vi "界面UI.vi"() -> ()   [LabVIEW 2016, in "科盛超标留样.lvlib"]
uses:
  <vilib>/Utility/miscctls.llb/LVPointTypeDef.ctl
  <vilib>/Utility/config.llb/NI_LVConfig.lvlib
  <vilib>/ptbypt/NI_PtbyPt.lvlib
panel:
  out "开关量3状态":T1
  out "开关量2状态":T2
  out "开关量1状态":T3
  out "元素":enum16{"open", "read", "write", "close"}(ring)
  out "供样完成":bool
  in  "返回":bool
  in  "查看记录":bool
  in  "当前解析模式":string(combo)
  in  "切换串口":bool
  out "查询系统状态":T4
  out "查询瓶记录":T5
  out "输出数组":T6(array[cluster])
  in  "留样命令":bool
  in  "供样命令":bool
  in  "触发采样":bool
  in  "查询系统状态":bool
  in  "远程取样":bool
  in  "复位指令":bool
  in  "查询瓶记录":bool
  in  "查询采样记录":bool
  in  "VISA resource name":refnum<visa-resource-name>="COM2" caption="VISA资源名称"
  in  "写入缓冲区":string
  out "读取缓冲区":string
  out "source":string
  out "通讯":bool
  # "启动顺序：先触发采样，然后仪器开始测试时发送供样命令此时采水到A/B桶，如果超标发送留样命令，如果在默认60分钟(可设置)后都没有接受到超标留样指令则自动排空。"
  # "科盛超标留样"
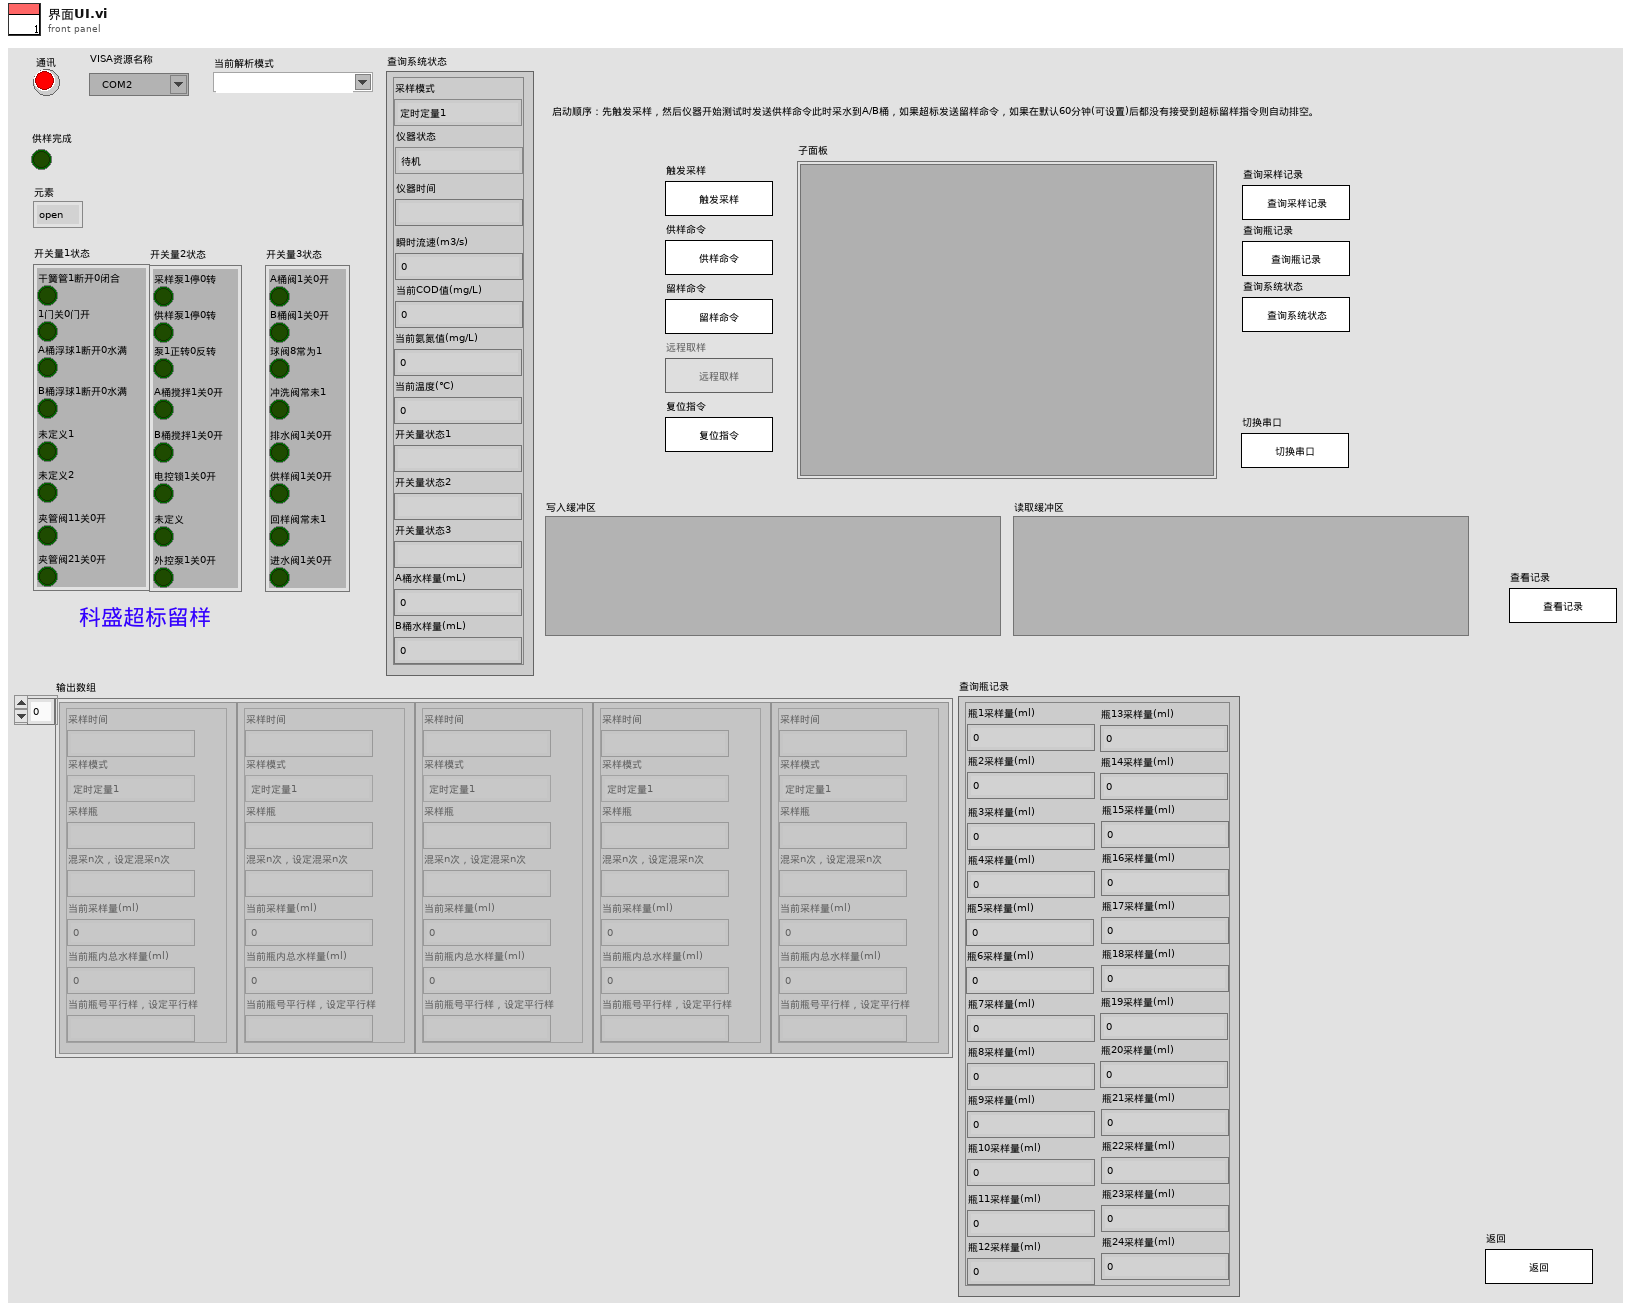
[diagram p1: front panel]
types:
  T1 = cluster{"A桶阀1关0开":bool, "B桶阀1关0开":bool, "球阀8常为1":bool, "冲洗阀常未1":bool, "排水阀1关0开":bool, "供样阀1关0开":bool, "回样阀常未1":bool, "进水阀1关0开":bool}
  T2 = cluster{"采样泵1停0转":bool, "供样泵1停0转":bool, "泵1正转0反转":bool, "A桶搅拌1关0开":bool, "B桶搅拌1关0开":bool, "电控锁1关0开":bool, "未定义":bool, "外控泵1关0开":bool}
  T3 = cluster{"干簧管1断开0闭合":bool, "1门关0门开":bool, "A桶浮球1断开0水满":bool, "B桶浮球1断开0水满":bool, "未定义1":bool, "未定义2":bool, "夹管阀11关0开":bool, "夹管阀21关0开":bool}
  T4 = cluster{"采样模式":enum16{"定时定量1", "定时定量2", "定流定量", "定时比例", "同步留样", "超标留样", "触发采样", "定时采样1", "定流供样", "定时采样2", "远程取样", "手动取样", "流量跟踪"}, "仪器状态":enum16{"待机", "运行中"}, "仪器时间":string, "瞬时流速(m3/s)":dbl, "当前COD值(mg/L)":dbl, "当前氨氮值(mg/L)":dbl, "当前温度(℃)":dbl, "开关量状态1":string, "开关量状态2":string, "开关量状态3":string, "A桶水样量(mL)":dbl, "B桶水样量(mL)":dbl}
  T5 = cluster{"瓶1采样量(ml)":dbl, "瓶2采样量(ml)":dbl, "瓶3采样量(ml)":dbl, "瓶4采样量(ml)":dbl, "瓶5采样量(ml)":dbl, "瓶6采样量(ml)":dbl, "瓶7采样量(ml)":dbl, "瓶8采样量(ml)":dbl, "瓶9采样量(ml)":dbl, "瓶10采样量(ml)":dbl, "瓶11采样量(ml)":dbl, "瓶12采样量(ml)":dbl, "瓶13采样量(ml)":dbl, "瓶14采样量(ml)":dbl, "瓶15采样量(ml)":dbl, "瓶16采样量(ml)":dbl, "瓶17采样量(ml)":dbl, "瓶18采样量(ml)":dbl, "瓶19采样量(ml)":dbl, "瓶20采样量(ml)":dbl, "瓶21采样量(ml)":dbl, "瓶22采样量(ml)":dbl, "瓶23采样量(ml)":dbl, "瓶24采样量(ml)":dbl}
  T6 = cluster{"采样时间":string, "采样模式":enum16{"定时定量1", "定时定量2", "定流定量", "定时比例", "同步留样", "超标留样", "触发采样", "定时采样1", "定流供样", "定时采样2", "远程取样", "手动取样", "流量跟踪"}, "采样瓶":string, "混采n次，设定混采n次":string, "当前采样量(ml)":dbl, "当前瓶内总水样量(ml)":dbl, "当前瓶号平行样，设定平行样":string}[]
  T7 = cluster{"STEP":enum16{"open", "read", "write", "close"}, "写入缓冲区":string}
  T8 = enum16{"触发采样", "供样命令", "留样命令", "远程取样", "复位指令", "查询采样记录", "查询瓶记录", "查询系统状态"}
  T9 = typedef "LVPointTypeDef.ctl" = cluster{"Horizontal":i16, "Vertical":i16}
  T10 = typedef "NI_LVConfig.lvlib/Config Data RefNum.ctl" = refnum<k1>
  T11 = cluster{"[0]":bool, "[1]":bool, "[2]":bool, "[3]":bool, "[4]":bool, "[5]":bool, "[6]":bool, "[7]":bool}
  T12 = cluster{"命令":string, "data":cluster{"starting address":u16, "coil values":bool[]}}
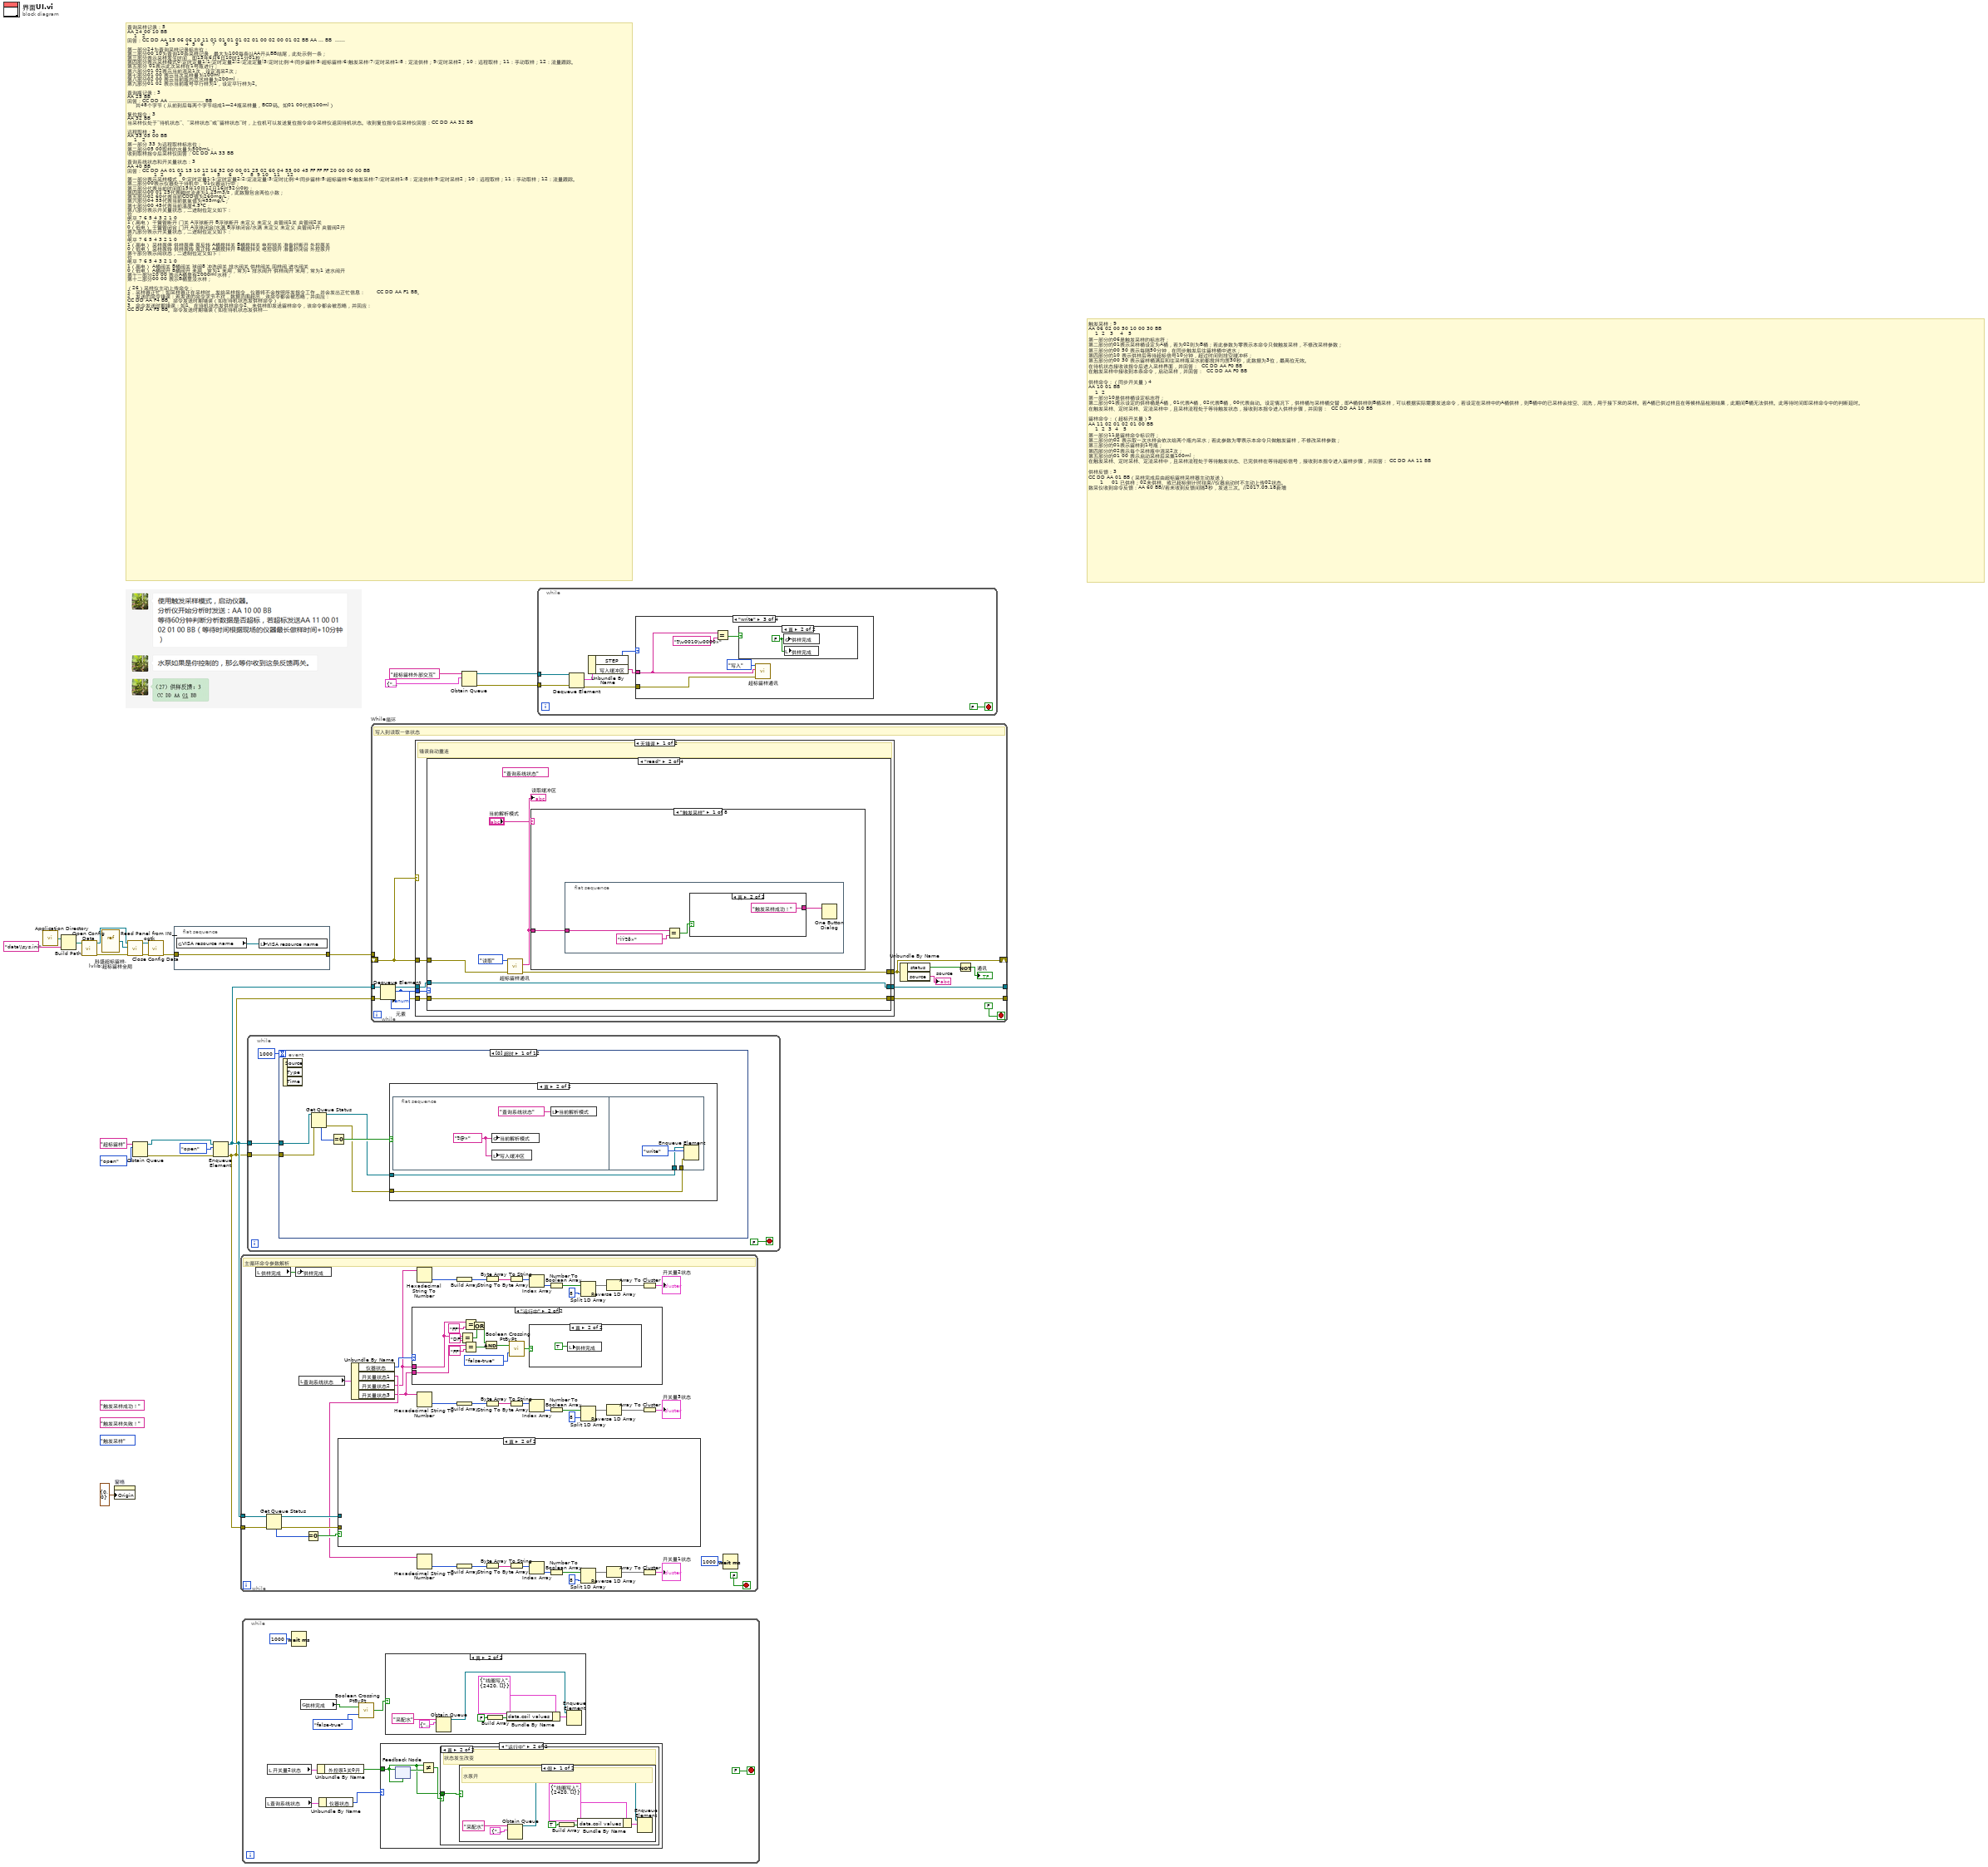
[diagram p0: block diagram]
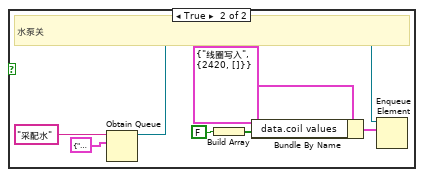
[diagram p4: hidden frame]
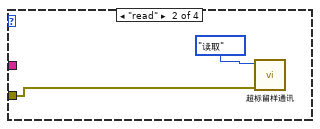
[diagram p7: hidden frame]
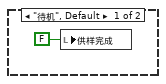
[diagram p10: hidden frame]
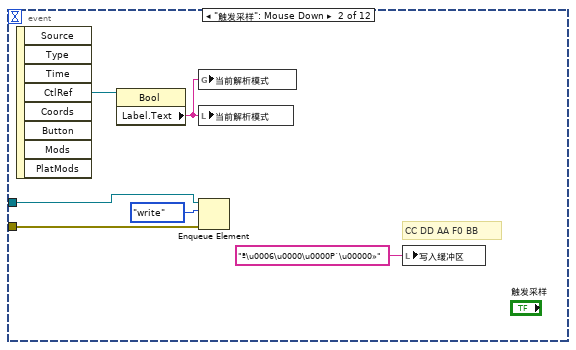
[diagram p14: hidden frame]
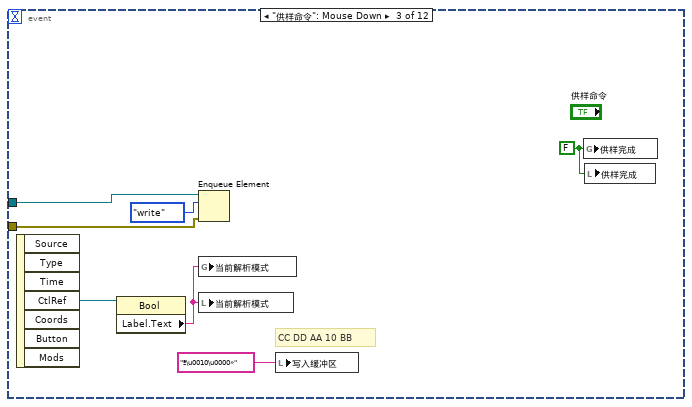
[diagram p15: hidden frame]
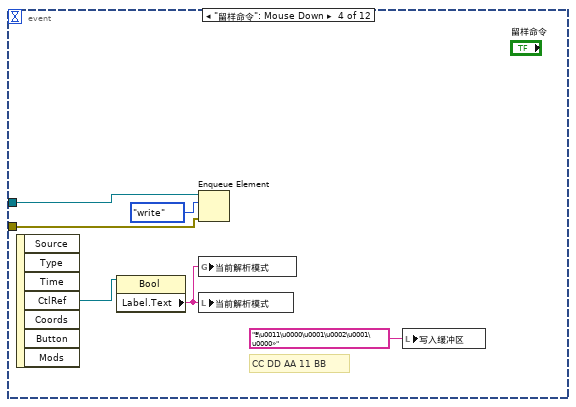
[diagram p16: hidden frame]
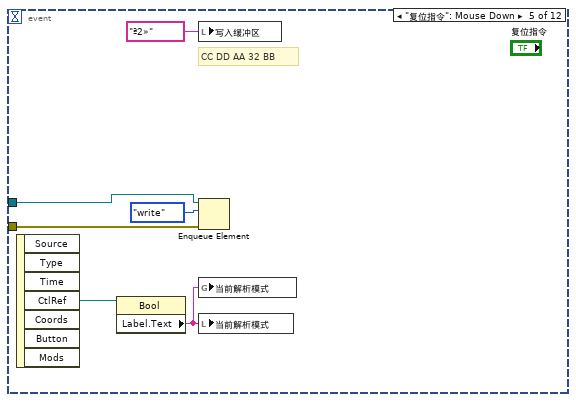
[diagram p17: hidden frame]
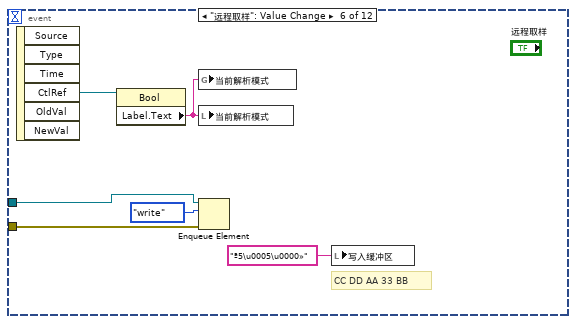
[diagram p18: hidden frame]
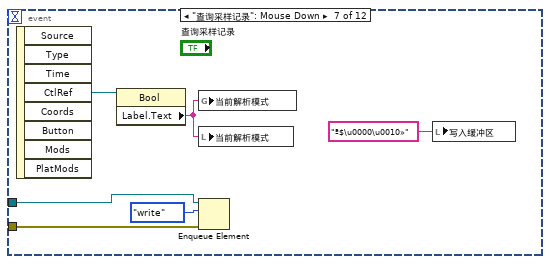
[diagram p19: hidden frame]
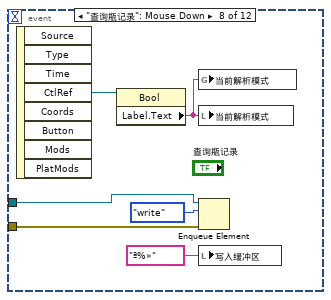
[diagram p20: hidden frame]
diagram:
  (unwired) "触发采样成功！" ("消息")
  (unwired) "触发采样失败！" ("消息")
  (unwired) T8."触发采样" ("功能输入")
  # "查询采样记录：5\nAA 24 00 10 BB\n    1   2\n回答：CC DD AA 15 06 06 10 11 01 01 01 01 02 01 00 02 00 01 02 BB AA ... BB  ......\n                       3          4  5   6     7     8     9\n第一部分24为查询采样记录标志位；\n第二部分00 10为查询10条采样记录，最大为100每条以AA开头BB结尾，此处示例一条；\n第三部分表示采样发生时间，即15年6月6日10时11分01秒；\n第四部分表示采样模式0:定时定量1;1:定时定量2;2:定流定量;3:定时比例;4:同步留样;5:超标留样;6:触发采样;7:定时采样1;8：定流供样；9:定时采样2；10：远程取样；11：手动取样；12：流量跟踪。\n第五部分 01表示此次采样在1号瓶进行；\n第六部分01 02表示当前混采1次，设定混采2次；\n第七部分01 00 表示当次采样量为100ml；\n第八部分02 00 表示当前瓶内总水样量为200ml；\n第九部分01 02 表示当前瓶号平行样为1，设定平行样为2。\n\n查询瓶记录：3\nAA 25 BB\n回答：CC DD AA ………………… BB\n     共48个字节（从前到后每两个字节组成1—24瓶采样量，BCD码。如01 00代表100ml）\n\n复位指令：3\nAA 32 BB\n当采样仪处于“待机状态”、“采样状态”或“留样状态”时，上位机可以发送复位指令命令采样仪返回待机状态。收到复位指令后采样仪回答：CC DD AA 32 BB\n\n远程取样：3\nAA 33 05 00 BB\n    1   2\n第一部分 33 为远程取样标志位；\n第二部分05 00取样的水量为500mL；\n收到取样指令后采样仪回答：CC DD AA 33 BB\n\n查询系统状态和开关量状态：3\nAA 40 BB\n回答：CC DD AA 01 01 15 10 12 16 52 00 00 01 25 02 60 04 55 00 45 FF FF FF 20 00 00 00 BB \n                1  2         3            4       5     6     7    8  9 10   11    12  \n第一部分表示采样模式，0:定时定量1;1:定时定量2;2:定流定量;3:定时比例;4:同步留样;5:超标留样;6:触发采样;7:定时采样1;8：定流供样;9:定时采样2；10：远程取样；11：手动取样；12：流量跟踪。\n第二部分00表示仪器处于待机中，01仪器运行中；\n第三部分代表当前时间即15年10月12日16时52分0秒； \n第四部分00 01 25代表瞬时流速为1.25m3/s，此数据包含两位小数；\n第五部分02 60代表当前COD值为260mg/L；\n第六部分04 55代表当前氨氮值为455mg/L；\n第七部分00 45代表当前温度4.5℃；\n第八部分表示开关量状态，二进制位定义如下：\n位\n电平\t7\t6\t5\t4\t3\t2\t1\t0\n1（高电）\t干簧管断开\t门关\tA浮球断开\tB浮球断开\t未定义\t未定义\t夹管阀1关\t夹管阀2关\n0（低电）\t干簧管闭合\t门开\tA浮球闭合/水满\tB浮球闭合/水满\t未定义\t未定义\t夹管阀1开\t夹管阀2开\n第九部分表示开关量状态，二进制位定义如下：\n位\n电平\t7\t6\t5\t4\t3\t2\t1\t0\n1（高电）\t采样泵停\t供样泵停\t泵反转\tA桶搅拌关\tB桶搅拌关\t电控锁关\t准备好断开\t外控泵关\n0（低电）\t采样泵转\t供样泵转\t泵正转\tA桶搅拌开\tB桶搅拌关\t电控锁开\t准备好闭合\t外控泵开\n第十部分表示阀状态，二进制位定义如下：\n位\n电平\t7\t6\t5\t4\t3\t2\t1\t0\n1（高电）\tA桶阀关\tB桶阀关\t球阀8\t冲洗阀关\t排水阀关\t供样阀关\t回样阀\t进水阀关\n0（低电）\tA桶阀开\tB桶阀开\t未用，常为1\t未用，常为1\t排水阀开\t供样阀开\t未用，常为1\t进水阀开\n第十一部分20 00 表示A桶里有2000ml水样；\n第十二部分00 00 表示B桶里没水样；\n\n（26）采样仪主动上传命令：\n1．采样器正忙：如采样器正在采样时，发给采样指令，仪器将不会按照所发指令工作，并会发出正忙信息：\t\t     CC DD AA F1 BB。\n2．发送的命令错误：若发送的命令字节不对，数据范围超出，该命令都会被忽略，并回应：\nCC DD AA F4 BB。命令发送时期错误（如在待机状态发供样命令），\n3．命令发送时期错误：如1、在待机状态发供样命令2、未供样即发送留样命令，该命令都会被忽略，并回应：\nCC DD AA F5 BB。命令发送时期错误（如在待机状态发供样命令），\n \t4．系统切换进入忙状态：仪器主动上传CC DD AA F6 BB。\n5．系统切换进入空闲状态：仪器主动上传CC DD AA F7 BB。"
  # "触发采样：9\nAA 06 02 00 50 10 00 30 BB\n    1  2   3    4   5         \n第一部分的06是触发采样的标志符；\n第二部分的01表示采样桶设定为A桶，若为02则为B桶；若此参数为零表示本命令只做触发采样，不修改采样参数；\n第三部分的00 50 表示每隔50分钟，在同步触发后往留样桶中进水；\n第四部分的10 表示供样后等待超标信号10分钟，超过时间则排空缓冲杯；\n第五部分的00 30 表示留样桶满后和往采样瓶采水前都搅拌均质30秒，此数据为3位，最高位无效。\n在待机状态接收该指令后进入采样界面，并回答：\t\tCC DD AA F0 BB\n在触发采样中接收到本条命令，启动采样，并回答：\t\tCC DD AA F0 BB\n\n供样命令：（同步开关量）4\nAA 10 01 BB\n    1  2  \n第一部分10是供样桶设定标志符；\n第二部分01表示设定的供样桶是A桶，01代表A桶，02代表B桶，00代表自动。设定情况下，供样桶与采样桶交替，即A桶供样则B桶采样，可以根据实际需要发送命令，若设定在采样中的A桶供样，则B桶中的已采样会排空、润洗，用于接下来的采样。若A桶已供过样且在等候样品检测结果，此期间B桶无法供样。此等待时间即采样命令中的判断延时。\n在触发采样、定时采样、定流采样中，且采样流程处于等待触发状态，接收到本指令进入供样步骤，并回答：\t\tCC DD AA 10 BB\n\n留样命令：（超标开关量）9\nAA 11 02 01 02 01 00 BB\n    1  2  3  4   5    \n第一部分11是留样命令标识符；\n第二部分的02 表示取一次水样会依次给两个瓶内采水；若此参数为零表示本命令只做触发留样，不修改采样参数；\n第三部分的01表示留样到1号瓶；\n第四部分的02表示每个采样瓶中混采2次；\n第五部分的01 00 表示启动采样后采集100ml；\n在触发采样、定时采样、定流采样中，且采样流程处于等待触发状态、已完供样在等待超标信号，接收到本指令进入留样步骤，并回答：\tCC DD AA 11 BB\n\n供样反馈：3\nCC DD AA 01 BB（采样完成后由超标留样采样器主动发送）\n  \t\t   1  \t\t\t01 已供样；02未供样、或已超标倒计时结束//仪器启动时不主动上传02状态。\n数采仪收到命令反馈：AA 60 BB//若未收到反馈间隔3秒，发送三次。//2017.09.18新增"
  n1 = call <vilib>:"Application Directory.vi"() -> ("Application Directory"=w14:path)
  n2 = Build Path(base path=w14, name or relative path="data\\sys.ini" ("名称或相对路径")) -> (appended path=w12:path)
  n3 = call <vilib>:"Open Config Data.vi"("configuration file path"=w12) -> ("error out"=w8:errorcluster, "refnum"=w11:T10)  [unwired: 8 in, 1 out]
  n4 = vi-ref "科盛超标留样.lvlib:超标留样全局.vi"() -> (w10:refnum<vi>)
  n5 = property on="窗格" class="Pane"("Origin"=T9 {"Horizontal"=0, "Vertical"=0} ("原点")) -> ()  [unwired: 2 in, 2 out]
  n6 = call <userlib>:"Read Panel from INI__ogtk.vi"("error in (no error)"=w8, "VI ref"=w10, "refnum"=w11) -> ("error out"=w7:errorcluster, "refnum out"=w9:T10)  [unwired: 7 in]
  n7 = Obtain Queue(name (unnamed)="超标留样" ("名称（未命名）"), element data type=enum16{"open", "read", "write", "close"}."open") -> (queue out=w20:refnum<queue>, error out=w19:errorcluster)  [unwired: 3 in, 1 out]
  n8 = call <vilib>:"Close Config Data.vi"("error in (no error)"=w7, "refnum"=w9) -> ("error out"=w6:errorcluster)  [unwired: 8 in, 1 out]
  n9 = flat-sequence {
    tunnel: w6 -> [w23]
    tunnel: [w23] -> w5
    frame #0 {
      n10 = global read "超标留样全局.vi" "VISA resource name"() -> (w24:refnum<visa-resource-name>)
      n11 = local write "VISA resource name"(w24) -> ()
    }
  }
  n12 = Enqueue Element(queue=w20, element=enum16{"open", "read", "write", "close"}."open", error in (no error)=w19) -> (queue out=w17:refnum<queue>, error out=w16:errorcluster)  [unwired: 1 in, 1 out]
  n13 = while {
    tunnel: w17 -> [w66]
    tunnel: w16 -> [w65]
    stop <- FALSE stop-if-true
    # "主循环命令参数解析"
    n14 = local read "供样完成"() -> (w37:bool)
    n15 = Get Queue Status(queue=w66, error in (no error)=w65) -> (queue out=w62:refnum<queue>, error out=w61:errorcluster, # elements in queue=w64:i32)  [unwired: 1 in, 5 out]
    n16 = global write "超标留样全局.vi" "供样完成"(w37) -> ()
    n17 = local read "查询系统状态"() -> (w60:T4)
    n18 = Equal To 0?(x=w64) -> (x = 0?=w63:bool)
    n19 = case shown="真" w63 {
      tunnel: w62 -> [_ _]
      tunnel: w61 -> [_ _]
      frame False {
      }
      frame True {
      }
    }
    n20 = Unbundle By Name(w60) -> ("仪器状态"=w59:enum16{"待机", "运行中"}, "开关量状态1"=w30:string, "开关量状态2"=w29:string, "开关量状态3"=w28:string)
    n21 = case shown="\"运行中\"" w59 {
      tunnel: w29 -> [_ w71]
      tunnel: w28 -> [_ w79]
      frame "待机", Default {
        n22 = local write "供样完成"(FALSE ("供样完成")) -> ()
      }
      frame "运行中" {
        n23 = Equal?(x=w71, y="DF" ("写入缓冲区")) -> (x = y?=w72:bool)
        n24 = Equal?(x=w71, y="FF" ("写入缓冲区")) -> (x = y?=w73:bool)
        n25 = Equal?(x=w79, y="FF" ("写入缓冲区")) -> (x = y?=w78:bool)
        n26 = Or(x=w73, y=w72) -> (x .or. y?=w74:bool)
        n27 = And(x=w74, y=w78) -> (x .and. y?=w77:bool)
        n28 = call <vilib>:"Boolean Crossing PtByPt.vi"("direction"=enum16{"either", "false-true", "true-false"}."false-true", "input"=w77) -> ("crossing"=w76:bool)  [unwired: 1 in]
        n29 = case shown="真" w76 {
          frame False {
          }
          frame True {
            n30 = local write "供样完成"(TRUE ("供样完成")) -> ()
          }
        }
      }
    }
    n31 = Hexadecimal String To Number(string=w29) -> (number=w33:u32)  [unwired: 2 in, 1 out]
    n32 = Hexadecimal String To Number(string=w28) -> (number=w32:u32)  [unwired: 2 in, 1 out]
    n33 = Hexadecimal String To Number(string=w30) -> (number=w36:u32)  [unwired: 2 in, 1 out]
    n34 = Build Array(w33) -> (w34:u32[])
    n35 = Build Array(w32) -> (w31:u32[])
    n36 = Build Array(w36) -> (w35:u32[])
    n37 = Byte Array To String(unsigned byte array=w34) -> (string=w26:string)
    n38 = Byte Array To String(unsigned byte array=w31) -> (string=w25:string)
    n39 = Byte Array To String(unsigned byte array=w35) -> (string=w27:string)
    n40 = String To Byte Array(string=w26) -> (unsigned byte array=w49:u8[])
    n41 = String To Byte Array(string=w25) -> (unsigned byte array=w48:u8[])
    n42 = String To Byte Array(string=w27) -> (unsigned byte array=w58:u8[])
    n43 = Index Array(array=w49) -> (element=w52:u8)  [unwired: 1 in]
    n44 = Index Array(array=w48) -> (element=w45:u8)  [unwired: 1 in]
    n45 = Index Array(array=w58) -> (element=w55:u8)  [unwired: 1 in]
    n46 = Number To Boolean Array(number=w52) -> (Boolean array=w53:bool[])
    n47 = Number To Boolean Array(number=w45) -> (Boolean array=w44:bool[])
    n48 = Number To Boolean Array(number=w55) -> (Boolean array=w54:bool[])
    n49 = Split 1D Array(array=w53, index=8 ("索引")) -> (first subarray=w50:bool[])  [unwired: 1 out]
    n50 = Split 1D Array(array=w44, index=8 ("索引")) -> (first subarray=w47:bool[])  [unwired: 1 out]
    n51 = Split 1D Array(array=w54, index=8 ("索引")) -> (first subarray=w57:bool[])  [unwired: 1 out]
    n52 = Reverse 1D Array(array=w50) -> (reversed array=w41:bool[])
    n53 = Reverse 1D Array(array=w47) -> (reversed array=w40:bool[])
    n54 = Reverse 1D Array(array=w57) -> (reversed array=w43:bool[])
    n55 = Array To Cluster(array=w41) -> (cluster=→"开关量2状态":T11)
    n56 = Array To Cluster(array=w40) -> (cluster=→"开关量3状态":T11)
    n57 = Array To Cluster(array=w43) -> (cluster=→"开关量1状态":T11)
    n58 = Wait (ms)(milliseconds to wait=u32 1000 ("等待时间（毫秒）")) -> ()  [unwired: 1 out]
  }
  n59 = while {
    stop <- FALSE stop-if-true
    n60 = local read "查询系统状态"() -> (w85:T4)
    n61 = local read "开关量2状态"() -> (w86:T2)
    n62 = Wait (ms)(milliseconds to wait=u32 1000 ("等待时间（毫秒）")) -> ()  [unwired: 1 out]
    n63 = global read "超标留样全局.vi" "供样完成"() -> (w88:bool)
    n64 = Unbundle By Name(w86) -> ("外控泵1关0开"=w83:bool)
    n65 = Unbundle By Name(w85) -> ("仪器状态"=w84:enum16{"待机", "运行中"})
    n66 = call <vilib>:"Boolean Crossing PtByPt.vi"("direction"=enum16{"either", "false-true", "true-false"}."false-true", "input"=w88) -> ("crossing"=w87:bool)  [unwired: 1 in]
    n67 = case shown="\"运行中\"" w84 {
      tunnel: w83 -> [_ w92]
      frame "待机", Default {
      }
      frame "运行中" {
        n68 = feedback-in #1(w92) -> ()
        n69 = feedback #1(w92) -> (w94:bool)
        n70 = Not Equal?(x=w92, y=w94) -> (x != y?=w93:bool)
        n71 = case shown="真" w93 {
          tunnel: w92 -> [_ w95]
          frame False {
          }
          frame True {
            # "状态发生改变"
            n72 = case shown="假" w95 {
              frame False {
                # "水泵开"
                n73 = Obtain Queue(name (unnamed)="采配水" ("名称（未命名）"), element data type=cluster{"命令":string, "数据":variant} {"命令"="", "数据"=variant}) -> (queue out=w96:refnum<queue>)  [unwired: 3 in, 2 out]
                n74 = Build Array(TRUE) -> (w99:bool[])
                n75 = Bundle By Name(cluster=T12 {"命令"="线圈写入", "data"={"starting address"=2420, "coil values"=[]}} ("元素"), "data.coil values"=w99) -> (w101:T12)
                n76 = Enqueue Element(queue=w96, element=w101) -> ()  [unwired: 2 in, 3 out]
              }
              frame True {
                # "水泵关"
                n77 = Obtain Queue(name (unnamed)="采配水" ("名称（未命名）"), element data type=cluster{"命令":string, "数据":variant} {"命令"="", "数据"=variant}) -> (queue out=w103:refnum<queue>)  [unwired: 3 in, 2 out]
                n78 = Build Array(FALSE) -> (w106:bool[])
                n79 = Bundle By Name(cluster=T12 {"命令"="线圈写入", "data"={"starting address"=2420, "coil values"=[]}} ("元素"), "data.coil values"=w106) -> (w108:T12)
                n80 = Enqueue Element(queue=w103, element=w108) -> ()  [unwired: 2 in, 3 out]
              }
            }
          }
        }
      }
    }
    n81 = case shown="真" w87 {
      frame False {
      }
      frame True {
        n82 = Obtain Queue(name (unnamed)="采配水" ("名称（未命名）"), element data type=cluster{"命令":string, "数据":variant} {"命令"="", "数据"=variant}) -> (queue out=w110:refnum<queue>)  [unwired: 3 in, 2 out]
        n83 = Build Array(FALSE) -> (w113:bool[])
        n84 = Bundle By Name(cluster=T12 {"命令"="线圈写入", "data"={"starting address"=2420, "coil values"=[]}} ("元素"), "data.coil values"=w113) -> (w115:T12)
        n85 = Enqueue Element(queue=w110, element=w115) -> ()  [unwired: 2 in, 3 out]
      }
    }
  }
  n86 = while {
    tunnel: w17 -> [w119]
    tunnel: w16 -> [w118]
    stop <- FALSE stop-if-true
    n87 = event shown="[0] 超时" {
      selector: _ -> [_ _ _ _ _ _ _ _ _ _ _ _]
      dyn-events: _ -> [_ _ _ _ _ _ _ _ _ _ _ _]
      timeout: 1000 -> [_ _ _ _ _ _ _ _ _ _ _ _]
      tunnel: w119 -> [w125 w138 w144 w151 w157 w163 w169 w175 w181 w183 _ _]
      tunnel: w118 -> [w124 w137 w145 w150 w156 w162 w168 w174 w180 w184 _ _]
      event Timeout {
        n88 = event-data() -> ()  [unwired: 1 in, 3 out]
        n89 = Get Queue Status(queue=w125, error in (no error)=w124) -> (queue out=w122:refnum<queue>, error out=w121:errorcluster, # elements in queue=w126:i32)  [unwired: 1 in, 5 out]
        n90 = Equal To 0?(x=w126) -> (x = 0?=w123:bool)
        n91 = case shown="真" w123 {
          tunnel: w122 -> [_ w128]
          tunnel: w121 -> [_ w127]
          frame False {
          }
          frame True {
            n92 = flat-sequence {
              tunnel: w128 -> [w132]
              tunnel: w127 -> [w131]
              frame #0 {
                w130 = "ª@»" ("写入缓冲区")
                n93 = global write "超标留样全局.vi" "当前解析模式"(w130) -> ()
                n94 = local write "写入缓冲区"(w130) -> ()
                n95 = local write "当前解析模式"("查询系统状态" ("当前解析模式")) -> ()
              }
              frame #1 {
                n96 = Enqueue Element(queue=w132, element=enum16{"open", "read", "write", "close"}."write" ("元素"), error in (no error)=w131) -> ()  [unwired: 1 in, 3 out]
              }
            }
          }
        }
      }
      event "触发采样": Mouse Down {
        # "CC DD AA F0 BB"
        n97 = event-data() -> ("CtlRef"=w136:refnum<vi>)  [unwired: 1 in, 7 out]
        n98 = property class="Bool"(reference=w136) -> ("Label.Text"=w134:string)  [unwired: 1 in, 2 out]
        n99 = global write "超标留样全局.vi" "当前解析模式"(w134) -> ()
        n100 = local write "当前解析模式"(w134) -> ()
        n101 = Enqueue Element(queue=w138, element=enum16{"open", "read", "write", "close"}."write" ("元素"), error in (no error)=w137) -> ()  [unwired: 1 in, 3 out]
        n102 = local write "写入缓冲区"("ª\u0006\u0000\u0000P`\u00000»" ("写入缓冲区")) -> ()
      }
      event "供样命令": Mouse Down {
        w140 = FALSE ("供样完成")
        # "CC DD AA 10 BB"
        n103 = event-data() -> ("CtlRef"=w143:refnum<vi>)  [unwired: 1 in, 6 out]
        n104 = property class="Bool"(reference=w143) -> ("Label.Text"=w141:string)  [unwired: 1 in, 2 out]
        n105 = Enqueue Element(queue=w144, element=enum16{"open", "read", "write", "close"}."write" ("元素"), error in (no error)=w145) -> ()  [unwired: 1 in, 3 out]
        n106 = global write "超标留样全局.vi" "当前解析模式"(w141) -> ()
        n107 = local write "当前解析模式"(w141) -> ()
        n108 = local write "写入缓冲区"("ª\u0010\u0000»" ("写入缓冲区")) -> ()
        n109 = global write "超标留样全局.vi" "供样完成"(w140) -> ()
        n110 = local write "供样完成"(w140) -> ()
      }
      event "留样命令": Mouse Down {
        # "CC DD AA 11 BB"
        n111 = event-data() -> ("CtlRef"=w149:refnum<vi>)  [unwired: 1 in, 6 out]
        n112 = property class="Bool"(reference=w149) -> ("Label.Text"=w147:string)  [unwired: 1 in, 2 out]
        n113 = Enqueue Element(queue=w151, element=enum16{"open", "read", "write", "close"}."write" ("元素"), error in (no error)=w150) -> ()  [unwired: 1 in, 3 out]
        n114 = global write "超标留样全局.vi" "当前解析模式"(w147) -> ()
        n115 = local write "当前解析模式"(w147) -> ()
        n116 = local write "写入缓冲区"("ª\u0011\u0000\u0001\u0002\u0001\u0000»" ("写入缓冲区")) -> ()
      }
      event "复位指令": Mouse Down {
        # "CC DD AA 32 BB"
        n117 = event-data() -> ("CtlRef"=w155:refnum<vi>)  [unwired: 1 in, 6 out]
        n118 = property class="Bool"(reference=w155) -> ("Label.Text"=w153:string)  [unwired: 1 in, 2 out]
        n119 = local write "写入缓冲区"("ª2»" ("写入缓冲区")) -> ()
        n120 = Enqueue Element(queue=w157, element=enum16{"open", "read", "write", "close"}."write" ("元素"), error in (no error)=w156) -> ()  [unwired: 1 in, 3 out]
        n121 = global write "超标留样全局.vi" "当前解析模式"(w153) -> ()
        n122 = local write "当前解析模式"(w153) -> ()
      }
      event "远程取样": Value Change {
        # "CC DD AA 33 BB"
        n123 = event-data() -> ("CtlRef"=w161:refnum<vi>)  [unwired: 1 in, 5 out]
        n124 = property class="Bool"(reference=w161) -> ("Label.Text"=w159:string)  [unwired: 1 in, 2 out]
        n125 = global write "超标留样全局.vi" "当前解析模式"(w159) -> ()
        n126 = local write "当前解析模式"(w159) -> ()
        n127 = Enqueue Element(queue=w163, element=enum16{"open", "read", "write", "close"}."write" ("元素"), error in (no error)=w162) -> ()  [unwired: 1 in, 3 out]
        n128 = local write "写入缓冲区"("ª5\u0005\u0000»" ("写入缓冲区")) -> ()
      }
      event "查询采样记录": Mouse Down {
        n129 = event-data() -> ("CtlRef"=w167:refnum<vi>)  [unwired: 1 in, 7 out]
        n130 = property class="Bool"(reference=w167) -> ("Label.Text"=w165:string)  [unwired: 1 in, 2 out]
        n131 = global write "超标留样全局.vi" "当前解析模式"(w165) -> ()
        n132 = local write "当前解析模式"(w165) -> ()
        n133 = Enqueue Element(queue=w169, element=enum16{"open", "read", "write", "close"}."write" ("元素"), error in (no error)=w168) -> ()  [unwired: 1 in, 3 out]
        n134 = local write "写入缓冲区"("ª$\u0000\u0010»" ("写入缓冲区")) -> ()
      }
      event "查询瓶记录": Mouse Down {
        n135 = event-data() -> ("CtlRef"=w173:refnum<vi>)  [unwired: 1 in, 7 out]
        n136 = property class="Bool"(reference=w173) -> ("Label.Text"=w171:string)  [unwired: 1 in, 2 out]
        n137 = global write "超标留样全局.vi" "当前解析模式"(w171) -> ()
        n138 = local write "当前解析模式"(w171) -> ()
        n139 = Enqueue Element(queue=w175, element=enum16{"open", "read", "write", "close"}."write" ("元素"), error in (no error)=w174) -> ()  [unwired: 1 in, 3 out]
        n140 = local write "写入缓冲区"("ª%»" ("写入缓冲区")) -> ()
      }
      event "查询系统状态": Mouse Down {
        n141 = event-data() -> ("CtlRef"=w179:refnum<vi>)  [unwired: 1 in, 7 out]
        n142 = property class="Bool"(reference=w179) -> ("Label.Text"=w177:string)  [unwired: 1 in, 2 out]
        n143 = global write "超标留样全局.vi" "当前解析模式"(w177) -> ()
        n144 = local write "当前解析模式"(w177) -> ()
        n145 = local write "写入缓冲区"("ª@»" ("写入缓冲区")) -> ()
        n146 = Enqueue Element(queue=w181, element=enum16{"open", "read", "write", "close"}."write" ("元素"), error in (no error)=w180) -> ()  [unwired: 1 in, 3 out]
      }
      event "切换串口": Value Change {
        n147 = flat-sequence {
          frame #0 {
            n148 = local read "VISA resource name"() -> (w186:refnum<visa-resource-name>)
            n149 = global write "超标留样全局.vi" "VISA resource name"(w186) -> ()
          }
          frame #1 {
            n150 = call <vilib>:"Application Directory.vi"() -> ("Application Directory"=w188:path)
            n151 = Build Path(base path=w188, name or relative path="data\\sys.ini" ("名称或相对路径")) -> (appended path=w189:path)
            n152 = call <vilib>:"Open Config Data.vi"("configuration file path"=w189) -> ("error out"=w193:errorcluster, "refnum"=w190:T10)  [unwired: 8 in, 1 out]
            n153 = vi-ref "科盛超标留样.lvlib:超标留样全局.vi"() -> (w191:refnum<vi>)
            n154 = call <userlib>:"Write Panel to INI__ogtk.vi"("error in (no error)"=w193, "VI ref"=w191, "refnum"=w190) -> ("error out"=w194:errorcluster, "refnum out"=w192:T10)  [unwired: 7 in]
            n155 = call <vilib>:"Close Config Data.vi"("error in (no error)"=w194, "refnum"=w192) -> ("error out"=w199:errorcluster, "file path"=w200:path)  [unwired: 8 in]
            n156 = Open/Create/Replace File(file path (use dialog)=w200, error in=w199) -> (refnum out=w196:refnum<file>, error out=w195:errorcluster)  [unwired: 4 in, 1 out]
            n157 = Flush File(refnum=w196, error in=w195) -> (refnum out=w197:refnum<file>, error out=w198:errorcluster)
            n158 = Close File(refnum=w197, error in=w198) -> ()  [unwired: 2 out]
          }
        }
        n159 = event-data() -> ()  [unwired: 1 in, 6 out]
        n160 = Enqueue Element(queue=w183, element=enum16{"open", "read", "write", "close"}."close" ("元素"), error in (no error)=w184) -> ()  [unwired: 1 in, 3 out]
      }
      event "查看记录": Value Change {
        n161 = event-data() -> ()  [unwired: 1 in, 6 out]
        n162 = property on="窗格" class="Pane"("Origin"=T9 {"Horizontal"=0, "Vertical"=628} ("原点")) -> ()  [unwired: 2 in, 2 out]
      }
      event "返回": Value Change {
        n163 = event-data() -> ()  [unwired: 1 in, 6 out]
        n164 = property on="窗格" class="Pane"("Origin"=T9 {"Horizontal"=0, "Vertical"=0} ("原点")) -> ()  [unwired: 2 in, 2 out]
      }
    }
  }
  n165 = while "While循环" {
    tunnel: w17 -> [w214]
    tunnel: w16 -> [w213]
    tunnel: [w209] -> _
    tunnel: [w208] -> _
    shift-right: [w204] -> _
    shift-left: _ -> [w203]
    tunnel: w5 -> [_]
    stop <- FALSE stop-if-true
    # "写入到读取一体状态"
    n166 = Dequeue Element(queue=w214, error in (no error)=w213) -> (queue out=w211:refnum<queue>, element=w212:enum16{"open", "read", "write", "close"}, error out=w210:errorcluster)  [unwired: 1 in, 1 out]
    "元素" <- w212
    n167 = case shown="无错误" w203 {
      tunnel: w212 -> [w222 _]
      tunnel: w211 -> [w221 w316]
      tunnel: w210 -> [w220 w315]
      tunnel: [w219 w309] -> w209
      tunnel: [w218 w308] -> w208
      tunnel: w203 -> [w217 w311]
      tunnel: [w216 w310] -> w204
      frame No Error {
        # "错误自动重连"
        n168 = case shown="\"read\"" w222 {
          tunnel: [w226 w233 w293 w305] -> w216
          tunnel: w221 -> [w225 w231 w298 w304]
          tunnel: w220 -> [w224 w230 w297 w303]
          tunnel: [w225 w231 w296 w301] -> w219
          tunnel: [w224 w230 w295 w300] -> w218
          tunnel: w217 -> [_ w234 w294 w307]
          frame "open", Default {
            (unwired) refnum<visa-resource-name> "COM2" ("VISA resource name")
            n169 = global write "超标留样全局.vi" "VISA resource name"("VISA resource name") -> ()
            n170 = call "超标留样通讯.vi"("VISA resource name"="VISA resource name", "功能输入"=enum16{"打开串口", "写入", "读取", "关闭串口"}."打开串口") -> ("error out"=w226:errorcluster)  [unwired: 7 in, 2 out]
          }
          frame "read" {
            (unwired) "查询系统状态" ("当前解析模式")
            n171 = call "超标留样通讯.vi"("error in (no error)"=w234, "功能输入"=enum16{"打开串口", "写入", "读取", "关闭串口"}."读取") -> ("error out"=w233:errorcluster, "读取缓冲区"=w229:string)  [unwired: 7 in, 1 out]
            "读取缓冲区" <- w229
            n172 = case shown="\"触发采样\"" "当前解析模式" {
              tunnel: w229 -> [w235 w242 w249 w256 w263 w270 w276 w282]
              frame "触发采样" {
                n173 = flat-sequence {
                  tunnel: w235 -> [w239]
                  frame #0 {
                    n174 = Equal?(x=w239, y="ÌÝªð»") -> (x = y?=w237:bool)
                    n175 = case shown="真" w237 {
                      tunnel: ["触发采样失败！" ("消息") "触发采样成功！" ("消息")] -> w236
                      frame False {
                      }
                      frame True {
                      }
                    }
                    n176 = One Button Dialog(message=w236) -> ()  [unwired: 1 in, 1 out]
                  }
                }
              }
              frame "供样命令" {
                n177 = flat-sequence {
                  tunnel: w242 -> [w246]
                  frame #0 {
                    n178 = Equal?(x=w246, y="ÌÝª\u0010»") -> (x = y?=w244:bool)
                    n179 = case shown="真" w244 {
                      tunnel: ["供样失败！" ("消息") "供样成功！" ("消息")] -> w243
                      frame False {
                      }
                      frame True {
                      }
                    }
                    n180 = One Button Dialog(message=w243) -> ()  [unwired: 1 in, 1 out]
                  }
                }
              }
              frame "留样命令", Default {
                n181 = flat-sequence {
                  tunnel: w249 -> [w253]
                  frame #0 {
                    n182 = Equal?(x=w253, y="ÌÝª\u0011»") -> (x = y?=w251:bool)
                    n183 = case shown="真" w251 {
                      tunnel: ["留样失败！" ("消息") "留样成功！" ("消息")] -> w250
                      frame False {
                      }
                      frame True {
                      }
                    }
                    n184 = One Button Dialog(message=w250) -> ()  [unwired: 1 in, 1 out]
                  }
                }
              }
              frame "复位指令" {
                n185 = flat-sequence {
                  tunnel: w256 -> [w260]
                  frame #0 {
                    n186 = Equal?(x=w260, y="ÌÝª2»") -> (x = y?=w258:bool)
                    n187 = case shown="真" w258 {
                      tunnel: ["复位失败！" ("消息") "复位成功！" ("消息")] -> w257
                      frame False {
                      }
                      frame True {
                      }
                    }
                    n188 = One Button Dialog(message=w257) -> ()  [unwired: 1 in, 1 out]
                  }
                }
              }
              frame "远程取样" {
                n189 = flat-sequence {
                  tunnel: w263 -> [w267]
                  frame #0 {
                    n190 = Equal?(x=w267, y="ÌÝª3»") -> (x = y?=w265:bool)
                    n191 = case shown="假" w265 {
                      tunnel: ["远程取样失败！" ("消息") "远程取样成功！" ("消息")] -> w264
                      frame False {
                      }
                      frame True {
                      }
                    }
                    n192 = One Button Dialog(message=w264) -> ()  [unwired: 1 in, 1 out]
                  }
                }
              }
              frame "查询采样记录" {
                n193 = flat-sequence {
                  tunnel: w270 -> [w275]
                  frame #0 {
                    n194 = call "科盛查询命令解析.vi"("解析参数选择"=enum16{"查询采样记录", "查询瓶记录", "查询系统状态"}."查询采样记录", "命令输入"=w275) -> ("Variant"=w273:variant)  [unwired: 9 in]
                    n195 = Variant To Data(type=T6 [] ("输出数组"), Variant=w273) -> (data=→"输出数组":T6)  [unwired: 1 in, 1 out]
                  }
                }
              }
              frame "查询瓶记录" {
                n196 = flat-sequence {
                  tunnel: w276 -> [w281]
                  frame #0 {
                    n197 = call "科盛查询命令解析.vi"("解析参数选择"=enum16{"查询采样记录", "查询瓶记录", "查询系统状态"}."查询瓶记录", "命令输入"=w281) -> ("Variant"=w279:variant)  [unwired: 9 in]
                    n198 = Variant To Data(type=T5 {"瓶1采样量(ml)"=0.0, "瓶2采样量(ml)"=0.0, "瓶3采样量(ml)"=0.0, "瓶4采样量(ml)"=0.0, "瓶5采样量(ml)"=0.0, "瓶6采样量(ml)"=0.0, "瓶7采样量(ml)"=0.0, "瓶8采样量(ml)"=0.0, "瓶9采样量(ml)"=0.0, "瓶10采样量(ml)"=0.0, "瓶11采样量(ml)"=0.0, "瓶12采样量(ml)"=0.0, "瓶13采样量(ml)"=0.0, "瓶14采样量(ml)"=0.0, "瓶15采样量(ml)"=0.0, "瓶16采样量(ml)"=0.0, "瓶17采样量(ml)"=0.0, "瓶18采样量(ml)"=0.0, "瓶19采样量(ml)"=0.0, "瓶20采样量(ml)"=0.0, "瓶21采样量(ml)"=0.0, "瓶22采样量(ml)"=0.0, "瓶23采样量(ml)"=0.0, "瓶24采样量(ml)"=0.0} ("查询瓶记录"), Variant=w279) -> (data=→"查询瓶记录":T5)  [unwired: 1 in, 1 out]
                  }
                }
              }
              frame "查询系统状态" {
                n199 = flat-sequence {
                  tunnel: w282 -> [w284]
                  frame #0 {
                    n200 = Equal?(x=w284, y="ÌÝª\u0001»") -> (x = y?=w283:bool)
                    n201 = case shown="真" w283 {
                      frame False {
                      }
                      frame True {
                        w290 = TRUE ("供样完成")
                        n202 = global write "超标留样全局.vi" "供样完成"(w290) -> ()
                        "供样完成" <- w290
                      }
                    }
                    n203 = call "科盛查询命令解析.vi"("解析参数选择"=enum16{"查询采样记录", "查询瓶记录", "查询系统状态"}."查询系统状态", "命令输入"=w284) -> ("Variant"=w288:variant)  [unwired: 9 in]
                    n204 = Variant To Data(type=T4 {"采样模式"=enum."定时定量1", "仪器状态"=enum."待机", "仪器时间"="", "瞬时流速(m3/s)"=0.0, "当前COD值(mg/L)"=0.0, "当前氨氮值(mg/L)"=0.0, "当前温度(℃)"=0.0, "开关量状态1"="", "开关量状态2"="", "开关量状态3"="", "A桶水样量(mL)"=0.0, "B桶水样量(mL)"=0.0} ("查询系统状态"), Variant=w288) -> (data=→"查询系统状态":T4)  [unwired: 1 in, 1 out]
                  }
                }
              }
            }
          }
          frame "write" {
            n205 = Enqueue Element(queue=w298, element=enum16{"open", "read", "write", "close"}."read" ("元素"), error in (no error)=w297) -> (queue out=w296:refnum<queue>, error out=w295:errorcluster)  [unwired: 1 in, 1 out]
            n206 = call "超标留样通讯.vi"("error in (no error)"=w294, "写入缓冲区"="写入缓冲区", "功能输入"=enum16{"打开串口", "写入", "读取", "关闭串口"}."写入") -> ("error out"=w293:errorcluster)  [unwired: 6 in, 2 out]
          }
          frame "close" {
            n207 = Enqueue Element(queue=w304, element=enum16{"open", "read", "write", "close"}."open" ("元素"), error in (no error)=w303) -> (queue out=w301:refnum<queue>, error out=w300:errorcluster)  [unwired: 1 in, 1 out]
            n208 = call "超标留样通讯.vi"("error in (no error)"=w307, "功能输入"=enum16{"打开串口", "写入", "读取", "关闭串口"}."关闭串口") -> ("error out"=w305:errorcluster)  [unwired: 7 in, 2 out]
          }
        }
      }
      frame Error {
        n209 = Flush Queue(queue=w316, error in (no error)=w315) -> (queue out=w314:refnum<queue>, error out=w313:errorcluster)  [unwired: 1 out]
        n210 = call <vilib>:"Clear Errors.vi"("error in (no error)"=w311) -> ("error out"=w310:errorcluster)  [unwired: 5 in, 1 out]
        n211 = Enqueue Element(queue=w314, element=enum16{"open", "read", "write", "close"}."close" ("元素"), error in (no error)=w313) -> (queue out=w309:refnum<queue>, error out=w308:errorcluster)  [unwired: 1 in, 1 out]
      }
    }
    n212 = Unbundle By Name(w204) -> ("status"=w206:bool, "source"=→"source":string)
    n213 = Not(x=w206) -> (.not. x?=→"通讯":bool)
  }
  n214 = Obtain Queue(name (unnamed)="超标留样外部交互" ("名称（未命名）"), element data type=T7 {"STEP"=enum."write", "写入缓冲区"="ª\u0006\u0000\u0000P`\u00000»"}) -> (queue out=w2:refnum<queue>, error out=w1:errorcluster)  [unwired: 3 in, 1 out]
  n215 = while {
    tunnel: w2 -> [w322]
    tunnel: w1 -> [w321]
    stop <- FALSE stop-if-true
    n216 = Dequeue Element(queue=w322, error in (no error)=w321) -> (element=w320:T7, error out=w318:errorcluster)  [unwired: 1 in, 2 out]
    n217 = Unbundle By Name(w320) -> ("STEP"=w319:enum16{"open", "read", "write", "close"}, "写入缓冲区"=w317:string)
    n218 = case shown="\"write\"" w319 {
      tunnel: w318 -> [_ w324 w329 _]
      tunnel: w317 -> [_ _ w327 _]
      frame "open", Default {
      }
      frame "read" {
        n219 = call "超标留样通讯.vi"("error in (no error)"=w324, "功能输入"=enum16{"打开串口", "写入", "读取", "关闭串口"}."读取") -> ()  [unwired: 7 in, 3 out]
      }
      frame "write" {
        n220 = Equal?(x=w327, y="ª\u0010\u0000»") -> (x = y?=w326:bool)
        n221 = case shown="真" w326 {
          frame False {
          }
          frame True {
            w331 = FALSE ("供样完成")
            n222 = global write "超标留样全局.vi" "供样完成"(w331) -> ()
            n223 = local write "供样完成"(w331) -> ()
          }
        }
        n224 = call "超标留样通讯.vi"("error in (no error)"=w329, "写入缓冲区"=w327, "功能输入"=enum16{"打开串口", "写入", "读取", "关闭串口"}."写入") -> ()  [unwired: 6 in, 3 out]
      }
      frame "close" {
      }
    }
  }
